vi "ShutDownDiag.vi"(10 "Caption.Text":string) -> (0 "ShutDownNOW?":bool caption="Shutdown?", 2 "Exit?":bool)   [LabVIEW 2017]
panel:
  in  "Exit":bool
  in  "ShutDown":bool caption="Power has been lost. Please restore power soon to avoid shutdown."
  # "LOSS OF POWER IN MACHINE"
  # "SHUTDOWN NOW"
  # "EXIT PROGRAM"
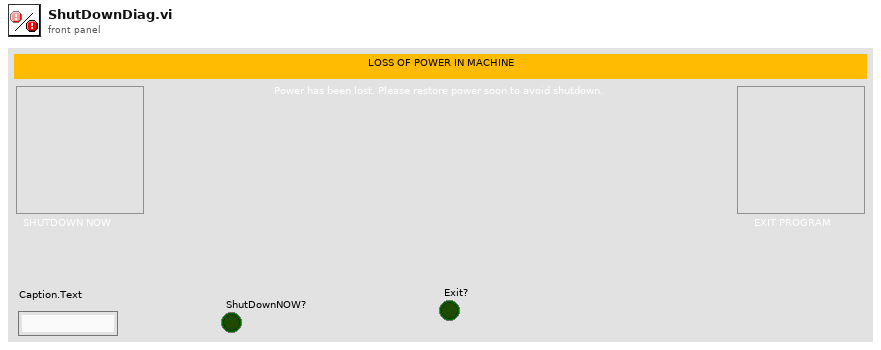
[diagram p1: front panel]
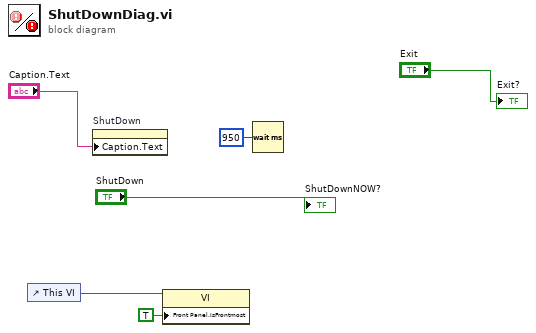
[diagram p0: block diagram]
diagram:
  n1 = control-ref of="This VI"() -> (w3:refnum<vi>)
  n2 = property on="ShutDown" class="Bool"("Caption.Text"="Caption.Text") -> ()  [unwired: 2 in, 2 out]
  n3 = property class="VI"(reference=w3, "Front Panel.IsFrontmost"=TRUE ("Front Panel Window:Is Frontmost")) -> ()  [unwired: 1 in, 2 out]
  n4 = Wait (ms)(milliseconds to wait=u32 950 ("millisecond multiple")) -> ()  [unwired: 1 out]
  "ShutDownNOW?" <- "ShutDown"
  "Exit?" <- "Exit"
